vi "ReadMasterStatus.vi"(11 "Active slaves":T2) -> (1 "done":bool, 3 "loop in progress":u8(slide) max=6 scale=0.0..6.0)   [LabVIEW 2018, in "MySharedVariables.lvlib"]
uses:
  MySharedVariables.lvlib
  MasterStatus.ctl
panel:
  out "MasterStatusShared":T1
  out "x*y":i32
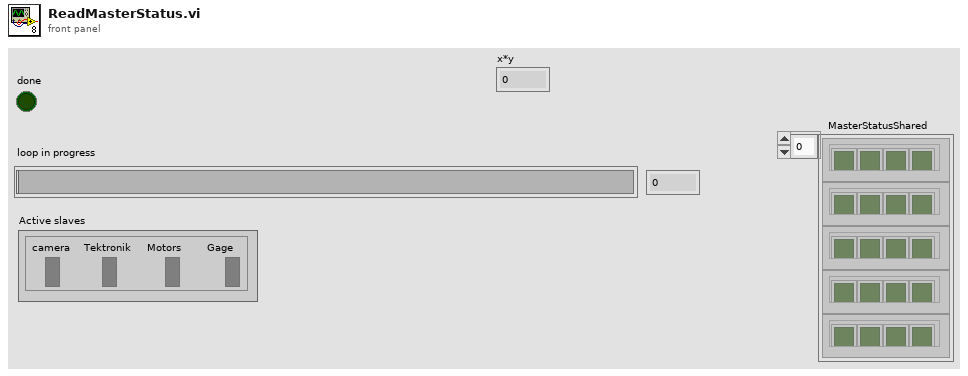
[diagram p1: front panel]
types:
  T1 = typedef "MySharedVariables.lvlib/MasterStatus.ctl" = cluster{"Camera done":bool, "Tektronik done":bool, "Motors done":bool, "Gage done":bool}[]
  T2 = cluster{"camera":bool, "Tektronik":bool, "Motors":bool, "Gage":bool}
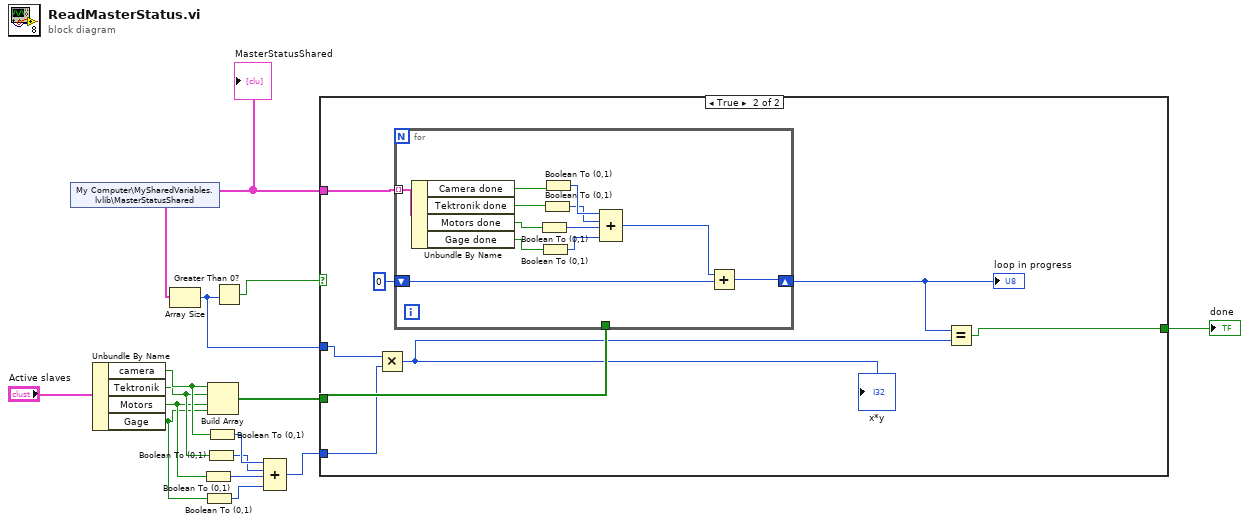
[diagram p0: block diagram]
diagram:
  n1 = shared-variable "My Computer\\MySharedVariables.lvlib\\MasterStatusShared"() -> (w14:T1)  [unwired: 1 in, 1 out]
  "MasterStatusShared" <- w14
  n2 = Unbundle By Name("Active slaves") -> ("camera"=w10:bool, "Tektronik"=w9:bool, "Motors"=w8:bool, "Gage"=w7:bool)
  n3 = Array Size(array=w14) -> (size(s)=w11:i32)
  n4 = Boolean To (0,1)(Boolean=w8) -> (0, 1=w4:i16)
  n5 = Boolean To (0,1)(Boolean=w7) -> (0, 1=w3:i16)
  n6 = Boolean To (0,1)(Boolean=w9) -> (0, 1=w5:i16)
  n7 = Boolean To (0,1)(Boolean=w10) -> (0, 1=w6:i16)
  n8 = Build Array(w10, w9, w8, w7) -> (w12:bool[])
  n9 = Greater Than 0?(x=w11) -> (x > 0?=w15:bool)
  n10 = Compound Arithmetic op=ADD(w6, w5, w4, w3) -> (w2:i16)
  n11 = case shown="True" w15 {
    tunnel: w14 -> [_ w19]
    tunnel: w12 -> [_ w22]
    tunnel: w11 -> [_ w21]
    tunnel: w2 -> [_ w20]
    tunnel: [_ w16] -> w1
    frame False {
    }
    frame True {
      n12 = Multiply(x=w21, y=w20) -> (x*y=w17:i32)
      "x*y" <- w17
      n13 = for {
        shift-right: [w35] -> w18
        shift-left: i16 0 -> [w34]
        tunnel: w22 -> [_]
        tunnel: w19 -> [w33] mode=indexing
        n14 = Unbundle By Name(w33) -> ("Camera done"=w28:bool, "Tektronik done"=w27:bool, "Motors done"=w26:bool, "Gage done"=w25:bool)
        n15 = Boolean To (0,1)(Boolean=w26) -> (0, 1=w30:i16)
        n16 = Boolean To (0,1)(Boolean=w25) -> (0, 1=w29:i16)
        n17 = Boolean To (0,1)(Boolean=w27) -> (0, 1=w31:i16)
        n18 = Boolean To (0,1)(Boolean=w28) -> (0, 1=w32:i16)
        n19 = Compound Arithmetic op=ADD(w32, w31, w30, w29) -> (w24:i16)
        n20 = Add(x=w24, y=w34) -> (x+y=w35:i16)
      }
      "loop in progress" <- w18
      n21 = Equal?(x=w18, y=w17) -> (x = y?=w16:bool)
    }
  }
  "done" <- w1
